vi "Home.vi"(8 "error in (no error)":errorcluster, 9 "Device and Axis":string, 11 "VISA resource name":refnum<visa-resource-name>) -> (0 "error out":errorcluster, 3 "VISA resource name out":refnum<visa-resource-name>)   [LabVIEW 2011, in "Zaber A Series.lvlib"]
doc: "Moves devices towards the motor end in order to provide a reference position for absolute movements. It's recommended that this sequence is run following the power on of the device, but doesn't need to be run again unless a) the power to the device is cycled, or b) the reference position is lost (device stalls). The VI will wait until the device has homed to continue.\n\nTo home a single device, specify the Device and Axis on the input.\n\nThis VI requires that the Initialize VI has been called with the same serial port."
uses:
  Zaber A Series.lvlib
  All Commands.ctl
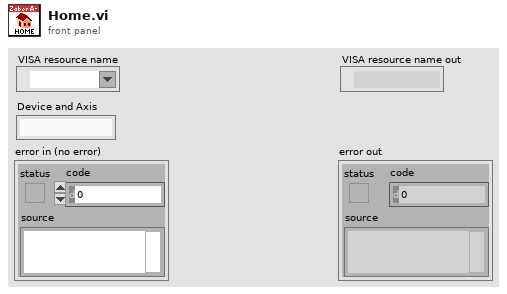
[diagram p1: front panel]
types:
  T1 = typedef "Zaber A Series.lvlib/All Commands.ctl" = string
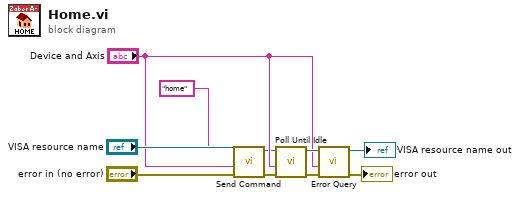
[diagram p0: block diagram]
diagram:
  n1 = call "Send Command.vi"("error in (no error)"="error in (no error)", "Device and Axis"="Device and Axis", "Command"=T1 "home" ("Command List"), "VISA resource name"="VISA resource name") -> ("error out"=w2:errorcluster, "VISA resource name out"=w1:refnum<visa-resource-name>)  [unwired: 3 in, 3 out]
  n2 = call "Poll Until Idle.vi"("error in (no error)"=w2, "Device and Axis"="Device and Axis", "VISA resource name"=w1) -> ("error out"=w10:errorcluster, "VISA resource name out"=w9:refnum<visa-resource-name>)  [unwired: 7 in]
  n3 = call "Error Query.vi"("error in (no error)"=w10, "Device and Axis"="Device and Axis", "VISA resource name"=w9) -> ("error out"=→"error out":errorcluster, "VISA resource name out"=→"VISA resource name out":refnum<visa-resource-name>)  [unwired: 5 in, 2 out]
